vi "Redis@Get__Parameter.vi"(1 "ParamterIn":string) -> (0 "ParamterOut":string)   [LabVIEW 2020]
panel:
  in  "Message=":string
  in  "TimeOut=":string(combo)
  in  "Variable=":string(combo)
  in  "Section":string(combo)
  in  "RedisSession":string(combo)
  in  "Confirm":bool
  # "RedisSession(,Variable=,TimeOut=XXX, Message=XXX)"
  # "@"
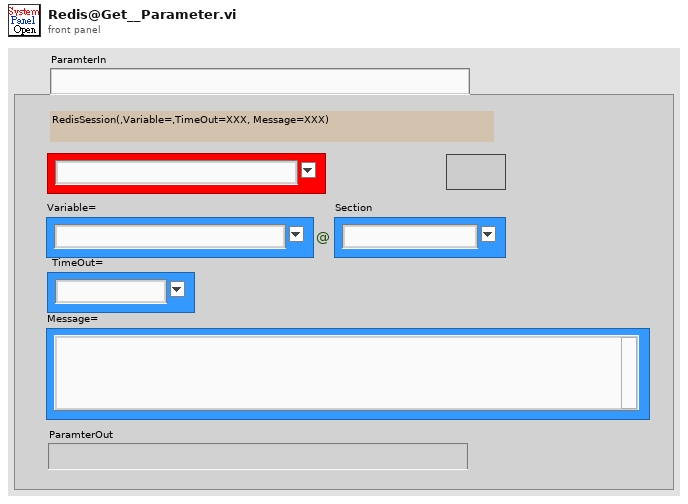
[diagram p1: front panel]
types:
  T1 = enum16{"Get", "Init", "Set", "Delete", "GetElement", "Inc", "Dec"}
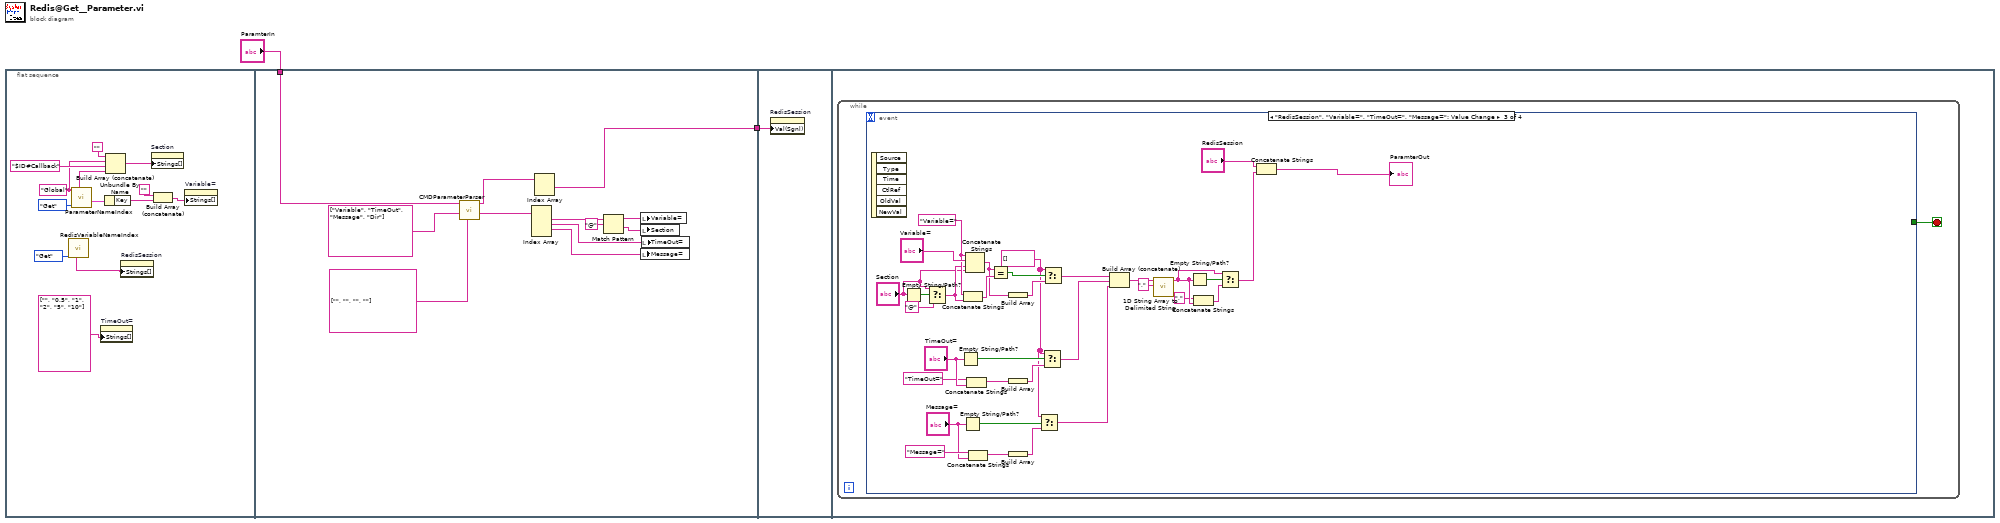
[diagram p0: block diagram]
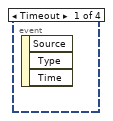
[diagram p2: hidden frame]
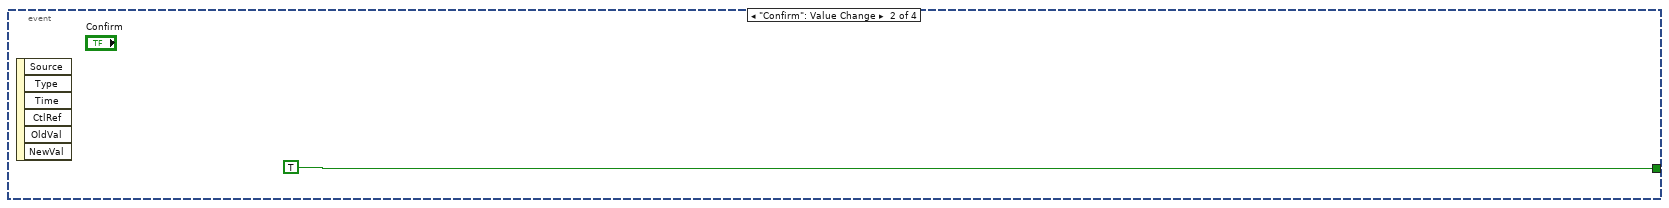
[diagram p3: hidden frame]
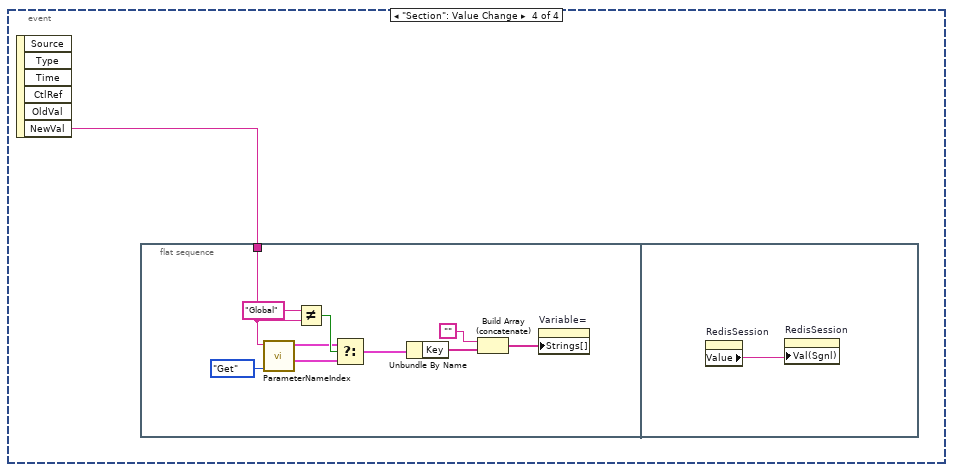
[diagram p4: hidden frame]
diagram:
  n1 = flat-sequence {
    tunnel: "ParamterIn" -> [w27]
    tunnel: [w23] -> w1
    tunnel: w1 -> [w28]
    frame #0 {
      w6 = "Global" ("VariableSection")
      n2 = call "RedisVariableNameIndex.vi"("OP"=enum16{"Add", "Init", "Get"}."Get") -> ("RedisSessionS"=w8:string[])  [unwired: 6 in, 4 out]
      n3 = call "ParameterNameIndex.vi"("OP"=T1."Get", "VariableSection"=w6) -> ("GlobalKeyValue"=w7:cluster{"Key":string[], "Value":string[]}, "SectionList"=w14:string[])  [unwired: 3 in, 5 out]
      n4 = property on="TimeOut=" class="CmbBox"("Strings[]"=string[] ["", "0.5", "1", "2", "5", "10"] ("Strings []")) -> ()  [unwired: 2 in, 2 out]
      n5 = Unbundle By Name(w7) -> ("Key"=w4:string[])
      n6 = Build Array (concatenate)("", w6, "$ID#Callback" ("VariableSection"), w14) -> (w13:string[])
      n7 = property on="RedisSession" class="CmbBox"("Strings[]"=w8) -> ()  [unwired: 2 in, 2 out]
      n8 = property on="Section" class="CmbBox"("Strings[]"=w13) -> ()  [unwired: 2 in, 2 out]
      n9 = Build Array (concatenate)("", w4) -> (w3:string[])
      n10 = property on="Variable=" class="CmbBox"("Strings[]"=w3) -> ()  [unwired: 2 in, 2 out]
    }
    frame #1 {
      n11 = call "CMDParameterParser.vi"("DeafultValues"=string[] ["", "", "", ""], "RequiredKeys"=string[] ["Variable", "TimeOut", "Message", "Dir"], "CMDParameter"=w27) -> ("KeyValues"=w22:string[], "Input"=w24:string[])  [unwired: 6 in, 1 out]
      n12 = Index Array(array=w22) -> (element #1=w21:string, element #2=w18:string, element #3=w17:string)  [unwired: 4 in, 1 out]
      n13 = Index Array(array=w24) -> (element #1=w23:string)  [unwired: 2 in, 1 out]
      n14 = Match Pattern(string=w21, regular expression="@") -> (before substring=w19:string, after substring=w16:string)  [unwired: 1 in, 2 out]
      n15 = local write "Variable="(w19) -> ()
      n16 = local write "Section"(w16) -> ()
      n17 = local write "Message="(w17) -> ()
      n18 = local write "TimeOut="(w18) -> ()
    }
    frame #2 {
      n19 = property on="RedisSession" class="CmbBox"("Val(Sgnl)"=w28) -> ()  [unwired: 2 in, 2 out]
    }
    frame #3 {
      n20 = while {
        stop <- w29 stop-if-true
        n21 = event shown="[2] \"RedisSession\", \"Variable=\", \"TimeOut=\", \"Message=\": Value Change" {
          selector: _ -> [_ _ _ _]
          dyn-events: _ -> [_ _ _ _]
          timeout: _ -> [_ _ _ _]
          tunnel: [_ TRUE _ _] -> w29
          event Timeout {
            n22 = event-data() -> ()  [unwired: 1 in, 3 out]
          }
          event "Confirm": Value Change {
            n23 = event-data() -> ()  [unwired: 1 in, 6 out]
          }
          event "RedisSession", "Variable=", "TimeOut=", "Message=": Value Change {
            w46 = string[] [] ("t")
            w59 = "Variable=" ("string")
            n24 = event-data() -> ()  [unwired: 1 in, 6 out]
            n25 = Empty String/Path?(string/path="Section") -> (empty?=w35:bool)
            n26 = Select(t="Section", s=w35, f="@") -> (s? t:f=w33:string)
            n27 = Empty String/Path?(string/path="TimeOut=") -> (empty?=w58:bool)
            n28 = Empty String/Path?(string/path="Message=") -> (empty?=w53:bool)
            n29 = Concatenate Strings(w59, w33) -> (w52:string)
            n30 = Concatenate Strings(w59, "Variable=", w33, "Section") -> (w36:string)
            n31 = Concatenate Strings("TimeOut=" ("string"), "TimeOut=") -> (w50:string)
            n32 = Concatenate Strings("Message=" ("string"), "Message=") -> (w48:string)
            n33 = Equal?(x=w36, y=w52) -> (x = y?=w60:bool)
            n34 = Build Array(w36) -> (w51:string[])
            n35 = Build Array(w50) -> (w49:string[])
            n36 = Build Array(w48) -> (w47:string[])
            n37 = Select(t=w46, s=w53, f=w47) -> (s? t:f=w43:string[])
            n38 = Select(t=w46, s=w58, f=w49) -> (s? t:f=w44:string[])
            n39 = Select(t=w46, s=w60, f=w51) -> (s? t:f=w45:string[])
            n40 = Build Array (concatenate)(w45, w44, w43) -> (w42:string[])
            n41 = call <vilib>:"1D String Array to Delimited String.vi"("delimiter"=",", "string array"=w42) -> ("delimited string"=w39:string)  [unwired: 9 in]
            n42 = Empty String/Path?(string/path=w39) -> (empty?=w40:bool)
            n43 = Concatenate Strings("," ("string"), w39) -> (w37:string)
            n44 = Select(t=w39, s=w40, f=w37) -> (s? t:f=w31:string)
            n45 = Concatenate Strings("RedisSession", w31) -> (→"ParamterOut":string)
          }
          event "Section": Value Change {
            n46 = event-data() -> ("NewVal"=w64:string)  [unwired: 1 in, 5 out]
            n47 = flat-sequence {
              tunnel: w64 -> [w73]
              frame #0 {
                n48 = call "ParameterNameIndex.vi"("OP"=T1."Get", "VariableSection"=w73) -> ("GlobalKeyValue"=w69:cluster{"Key":string[], "Value":string[]}, "SectionKeyValue"=w70:cluster{"Key":string[], "Value":string[]})  [unwired: 3 in, 5 out]
                n49 = Not Equal?(x="Global", y=w73) -> (x != y?=w71:bool)
                n50 = Select(t=w70, s=w71, f=w69) -> (s? t:f=w68:cluster{"Key":string[], "Value":string[]})
                n51 = Unbundle By Name(w68) -> ("Key"=w67:string[])
                n52 = Build Array (concatenate)("", w67) -> (w65:string[])
                n53 = property on="Variable=" class="CmbBox"("Strings[]"=w65) -> ()  [unwired: 2 in, 2 out]
              }
              frame #1 {
                n54 = property on="RedisSession" class="CmbBox"() -> ("Value"=w75:string)  [unwired: 2 in, 2 out]
                n55 = property on="RedisSession" class="CmbBox"("Val(Sgnl)"=w75) -> ()  [unwired: 2 in, 2 out]
              }
            }
          }
        }
      }
    }
  }
